vi "Msg Output Indicator To Control.vi"(10 "Msg Output All Terminals":i32[](array[numeric])) -> (2 "Msg Output All Terminals (For Init Msg Output.vi)":i32[](array[numeric]))   [LabVIEW 2025, in "_Msg Rescript.lvlib" / "_Msg Rescript.lvclass"]
uses:
  _Msg Rescript.lvclass
  _Msg Rescript.lvclass/_Msg Rescript.ctl
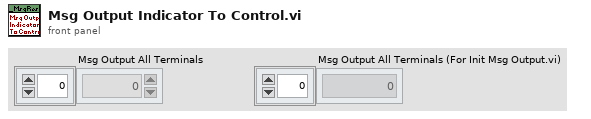
[diagram p1: front panel]
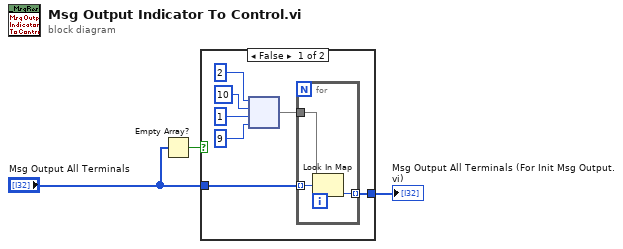
[diagram p0: block diagram]
diagram:
  n1 = Empty Array?(array="Msg Output All Terminals") -> (empty?=w1:bool)
  n2 = case shown="False" w1 {
    tunnel: [w6 w14] -> w3
    tunnel: "Msg Output All Terminals" -> [w5 w14]
    frame False {
      n3 = node(2 ("Numeric"), 10 ("Numeric"), 1 ("Numeric"), 9 ("Numeric")) -> (w4:map{i32, i32})
      n4 = for {
        tunnel: [w11] -> w6 mode=indexing
        tunnel: w5 -> [w12] mode=indexing
        tunnel: w4 -> [w13]
        n5 = Look In Map(map=w13, key=w12) -> (value=w11:i32)  [unwired: 1 in, 1 out]
      }
    }
    frame True {
    }
  }
  "Msg Output All Terminals (For Init Msg Output.vi)" <- w3
